vi "Draw Background.vi"(7 "Layout":T1) -> (8 "2D Picture":picture)   [LabVIEW 2015, in "HRTF Config.xctl"]
uses:
  HRTF Config.xctl
  Layout.ctl
  Item.ctl
panel:
  in  "Width":u16=3
  in  "color(black)":u32(colorbox)
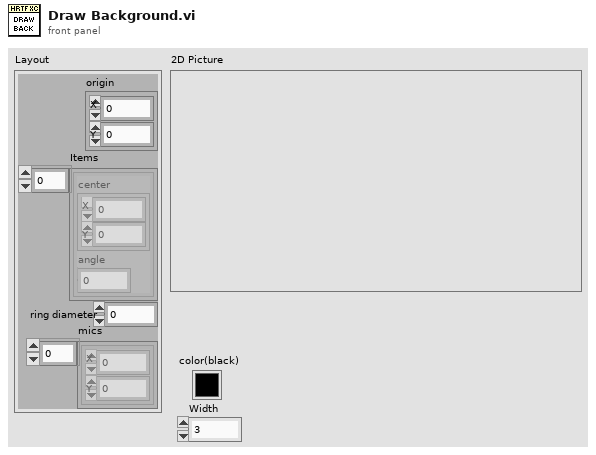
[diagram p1: front panel]
types:
  T1 = typedef "HRTF Config.xctl/Layout.ctl" = cluster{"origin":cluster{"X":i32, "Y":i32}, "Items":T2[], "ring diameter":i32, "mics":cluster{"X":i32, "Y":i32}[]}
  T2 = typedef "HRTF Config.xctl/Item.ctl" = cluster{"center":cluster{"X":i32, "Y":i32}, "angle":dbl}
  T3 = cluster{"Width":u16, "Style":enum32{"Solid", "Dash", "Dot", "DashDot", "DashDotDot"}}
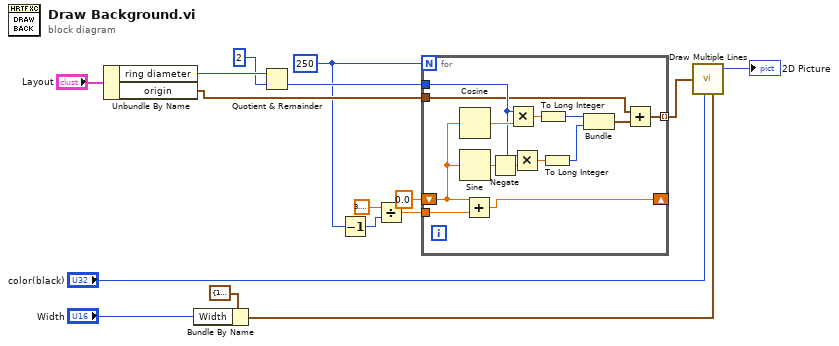
[diagram p0: block diagram]
diagram:
  w5 = 250
  n1 = Unbundle By Name("Layout") -> ("ring diameter"=w13:i32, "origin"=w9:cluster{"X":i32, "Y":i32})
  n2 = Bundle By Name(cluster=T3 {"Width"=1, "Style"=enum."Solid"} ("pen"), "Width"="Width") -> (w3:T3)
  n3 = Quotient & Remainder(x=w13, y=2) -> (floor(x/y)=w8:i32)  [unwired: 1 out]
  n4 = Decrement(x=w5) -> (x-1=w6:i32)
  n5 = Divide(x=3.141592653589793, y=w6) -> (x/y=w4:dbl)
  n6 = for {
    N: w5 -> [_]
    tunnel: w9 -> [w20]
    shift-right: [w30] -> _
    shift-left: 0.0 -> [w17]
    tunnel: w4 -> [w29]
    tunnel: w8 -> [w25]
    tunnel: [w18] -> w7 mode=indexing
    n7 = Cosine(x=w17) -> (cos(x)=w28:dbl)
    n8 = Sine(x=w17) -> (sin(x)=w24:dbl)
    n9 = Add(x=w17, y=w29) -> (x+y=w30:dbl)
    n10 = Negate(x=w24) -> (-x=w19:dbl)
    n11 = Multiply(x=w25, y=w28) -> (x*y=w27:dbl)
    n12 = Multiply(x=w25, y=w19) -> (x*y=w26:dbl)
    n13 = To Long Integer(number=w27) -> (32bit integer=w23:i32)
    n14 = To Long Integer(number=w26) -> (32bit integer=w22:i32)
    n15 = Bundle(w23, w22) -> (w21:cluster{i32, i32})  [unwired: 1 in]
    n16 = Add(x=w20, y=w21) -> (x+y=w18:cluster{i32, i32})
  }
  n17 = call <vilib>:"Draw Multiple Lines.vi"("line endpoints"=w7, "color(black)"="color(black)", "pen"=w3) -> ("new picture"=→"2D Picture":picture)  [unwired: 6 in]
